vi "CRYUnflatten Limits.vi"(9 "Step Name":string, 11 "Unflatten Limits":string) -> (0 "Error?":bool, 2 "Limits":T1={"Name"="", "Tolerance"=2, "X Axis"=1, "Limits"=2, "Upper Limit"=[{100.0, 1.0}, {1000.0, 1.0}], "Align Ref"={1000.0, 0.0}, "Lower Limit"=[{100.0, -1.0}, {1000.0, -1.0}], "Y data"=1, "Y unit"="(und)", "Y dB ref"=1.0, "Curve Names"=[], "Y-Resolution"=1, "Type"=1, "x float"=FALSE, "X min-max-step"={"Limit X Offset Min"=0.9, "Limit X Offset Max"=1.1, "Limit X Offset Step Size"=1.01}, "magn/phase"=1, "Upper Limit Type"=0, "Lower Limit Type"=0, "Lim Curve axis up"=1, "Lim Curve axis lo"=1, "Data Selection Upper"=1, "Data Selection Lower"=1, "X-Resolution"=1, "Output failed point curves?"=FALSE, "X data"=1, "X unit"="(und)", "X dB ref"=1.0, "X-Y Graph Set-up"="", "Tab Value"=enum."Parameters", "Help"="", "X Up Val"=0.0, "Y Up Val"=0.0, "X Low Val"=0.0, "Y Low Val"=0.0, "Up Limit Val"=0.0, "Low Limit Val"=0.0, "bAdd DataName"=FALSE, "Custom Name"=""} {"X data" items=["dB", "Lin"]; "Data Selection Lower" items=["Single Values", "Curves", "Waveforms"]; "Data Selection Upper" items=["Single Values", "Curves", "Waveforms"]; "Lim Curve axis lo" items=["x", "y", "z"]; "Lim Curve axis up" items=["x", "y", "z"]; "Lower Limit Type" items=["User Defined", "Memory List"]; "Upper Limit Type" items=["User Defined", "Memory List"]; "Type" items=["Single Value", "Curve", "Waveforms", "Voltmeter"]; "Y data" items=["dB", "Lin"]; "Limits" items=["Upper Only", "Lower Only", "Upper & Lower"]; "X Axis" items=["Linear", "Logarithmic"]; "Tolerance" items=["Individual Points", "Absolute Limits", "Floating Limits", "Floating Data", "Aligned Limits", "Aligned Data"]}, 3 "Header info":T2={"Data type"="Data            ", "Version"=1, "Dimensions"=0})   [LabVIEW 2013]
uses:
  Typedef Control/CRYLimits.ctl
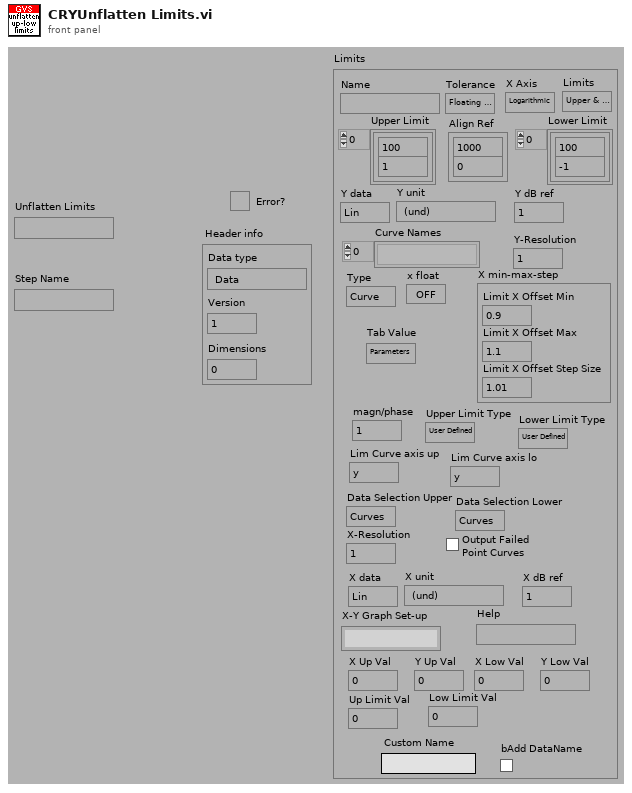
[diagram p1: front panel]
types:
  T1 = typedef "CRYLimits.ctl" = cluster{"Name":string, "Tolerance":u16, "X Axis":u16, "Limits":u16, "Upper Limit":cluster{dbl, dbl}[], "Align Ref":cluster{dbl, dbl}, "Lower Limit":cluster{dbl, dbl}[], "Y data":u16, "Y unit":string, "Y dB ref":dbl, "Curve Names":string[], "Y-Resolution":u8, "Type":u16, "x float":bool, "X min-max-step":cluster{"Limit X Offset Min":dbl, "Limit X Offset Max":dbl, "Limit X Offset Step Size":dbl}, "magn/phase":u16, "Upper Limit Type":u16, "Lower Limit Type":u16, "Lim Curve axis up":u16, "Lim Curve axis lo":u16, "Data Selection Upper":u16, "Data Selection Lower":u16, "X-Resolution":u8, "Output failed point curves?":bool, "X data":u16, "X unit":string, "X dB ref":dbl, "X-Y Graph Set-up":string, "Tab Value":enum32{"Data", "Parameters"}, "Help":string, "X Up Val":dbl, "Y Up Val":dbl, "X Low Val":dbl, "Y Low Val":dbl, "Up Limit Val":dbl, "Low Limit Val":dbl, "bAdd DataName":bool, "Custom Name":string}
  T2 = cluster{"Data type":string, "Version":u16, "Dimensions":u8}
  T3 = cluster{"Name":string, "Tolerance":u16, "X Axis":u16, "Limits":u16, "Upper Limit":cluster{dbl, dbl}[], "Align Ref":cluster{dbl, dbl}, "Lower Limit":cluster{dbl, dbl}[], "Y data":u16, "Y unit":string, "Y dB ref":dbl, "Curve Names":string[], "Y-Resolution":u8, "Type":u16, "x float":bool, "X min-max-step":cluster{"Limit X Offset Min":dbl, "Limit X Offset Max":dbl, "Limit X Offset Step Size":dbl}, "magn/phase":u16, "Upper Limit Type":u16, "Lower Limit Type":u16, "Lim Curve axis up":u16, "Lim Curve axis lo":u16, "Data Selection Upper":u16, "Data Selection Lower":u16, "X-Resolution":u8, "Output failed point curves?":bool, "X data":u16, "X unit":string, "X dB ref":dbl, "X-Y Graph Set-up":string, "Tab Value":enum32{"Data", "Parameters"}, "Help":string, "X Up Val":dbl, "Y Up Val":dbl, "X Low Val":dbl, "Y Low Val":dbl, "Up Limit Val":dbl, "Low Limit Val":dbl, "bAdd DataName":bool, "Custom Name":string}
  T4 = cluster{"unsigned byte array[0]":u8, "unsigned byte array[1]":u8, "unsigned byte array[2]":u8}
  T5 = cluster{"Name":string, "Tolerance":u16, "X Axis":u16, "Limits":u16, "Upper Limit":cluster{dbl, dbl}[], "Align Ref":cluster{dbl, dbl}, "Lower Limit":cluster{dbl, dbl}[], "Y data":u16, "Y unit":string, "Y dB ref":dbl, "Curve Names":string[], "Y-Resolution":u8, "Type":u16, "x float":bool, "X min-max-step":cluster{"Limit X Offset Min":dbl, "Limit X Offset Max":dbl, "Limit X Offset Step Size":dbl}, "magn/phase":u16, "Upper Limit Type":u16, "Lower Limit Type":u16, "Lim Curve axis up":u16, "Lim Curve axis lo":u16, "Data Selection Upper":u16, "Data Selection Lower":u16, "X-Resolution":u8, "Output failed point curves?":bool, "X data":u16, "X unit":string, "X dB ref":dbl, "X-Y Graph Set-up":string, "Tab Value":enum32{"Data", "Parameters", "Help"}}
  T6 = cluster{"Limit X Offset Min":dbl, "Limit X Offset Max":dbl, "Limit X Offset Step Size":dbl}
  T7 = cluster{"Name":string, "Tolerance":u16, "X Axis":u16, "Limits":u16, "Upper Limit":cluster{dbl, dbl}[], "Align Ref":cluster{dbl, dbl}, "Lower Limit":cluster{dbl, dbl}[], "Y data":u16, "Y unit":string, "Y dB ref":dbl, "Curve Names":string[], "Y-Resolution":u8, "Type":u16, "x float":bool, "X min-max-step":cluster{"Limit X Offset Min":dbl, "Limit X Offset Max":dbl, "Limit X Offset Step Size":dbl}, "magn/phase":u16, "Upper Limit Type":u16, "Lower Limit Type":u16, "Lim Curve axis up":u16, "Lim Curve axis lo":u16, "Data Selection Upper":u16, "Data Selection Lower":u16, "X-Resolution":u8, "Output failed point curves?":bool, "X data":u16, "X unit":string, "X dB ref":dbl, "X-Y Graph Set-up":string, "Tab Value":enum32{"Data", "Parameters"}, "Help":string}
  T8 = cluster{"Name":string, "Tolerance":u16, "X Axis":u16, "Limits":u16, "Upper Limit":cluster{dbl, dbl}[], "Align Ref":cluster{dbl, dbl}, "Lower Limit":cluster{dbl, dbl}[], "Y data":u16, "Y unit":string, "Y dB ref":dbl, "Curve Names":string[], "Y-Resolution":u8, "Type":u16, "x float":bool, "X min-max-step":cluster{"Limit X Offset Min":dbl, "Limit X Offset Max":dbl, "Limit X Offset Step Size":dbl}, "magn/phase":u16, "Upper Limit Type":u16, "Lower Limit Type":u16, "Lim Curve axis up":u16, "Lim Curve axis lo":u16, "Data Selection Upper":u16, "Data Selection Lower":u16, "X-Resolution":u8, "Output failed point curves?":bool, "X data":u16, "X unit":string, "X dB ref":dbl, "X-Y Graph Set-up":string, "Tab Value":enum32{"Data", "Parameters"}, "Help":string, "X Up Val":dbl, "Y Up Val":dbl, "X Low Val":dbl, "Y Low Val":dbl, "Up Limit Val":dbl, "Low Limit Val":dbl}
  T9 = cluster{"substring":string, u16, "unsigned byte array[2]":u8}
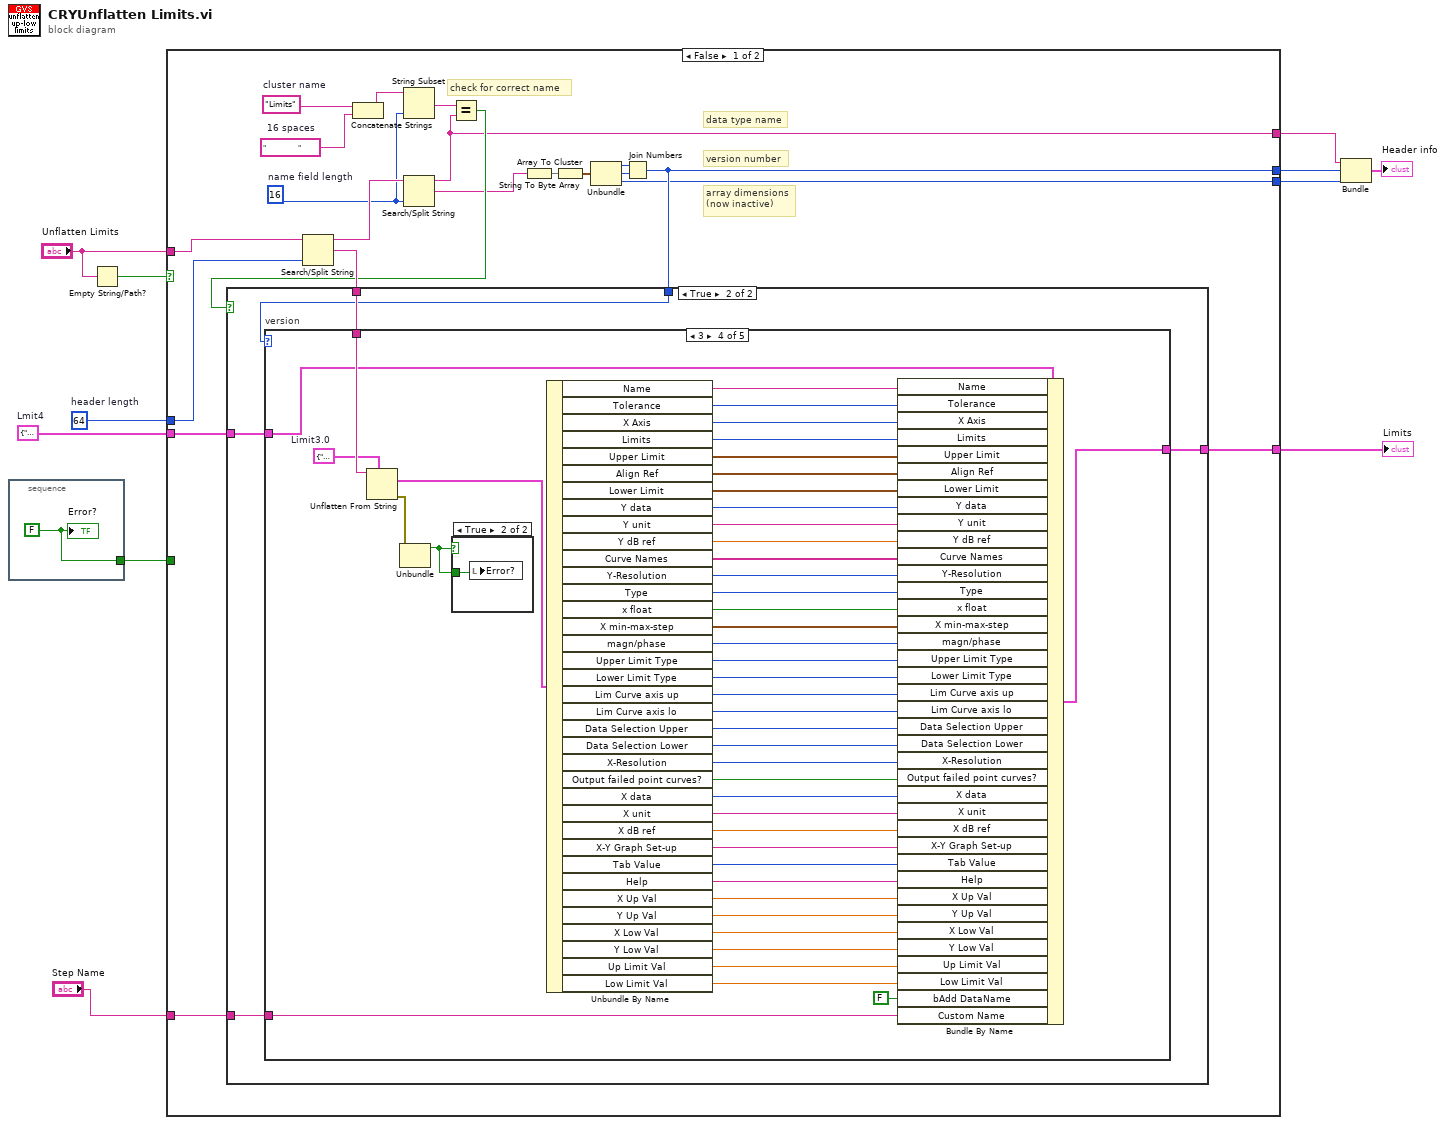
[diagram p0: block diagram]
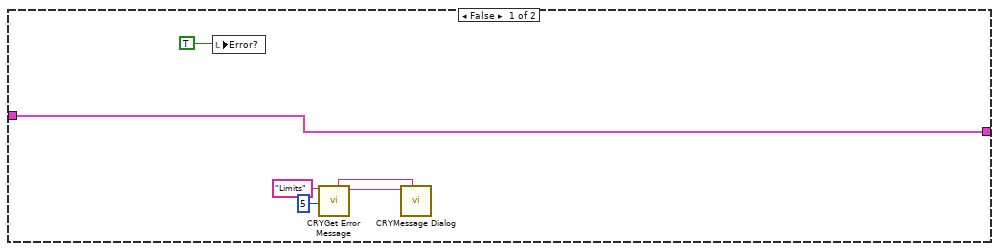
[diagram p2: hidden frame]
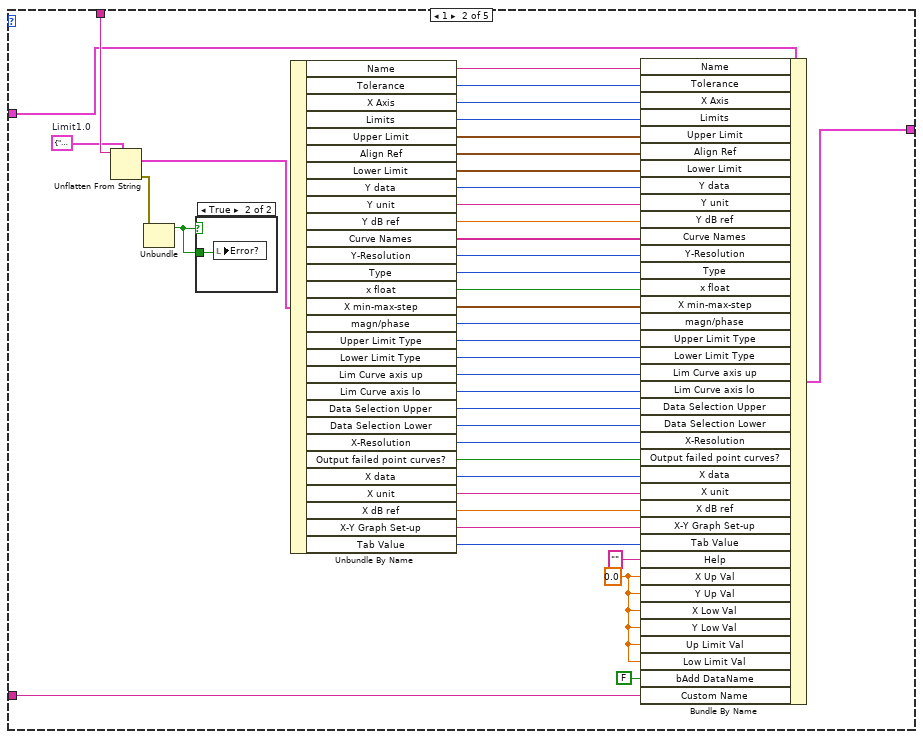
[diagram p4: hidden frame]
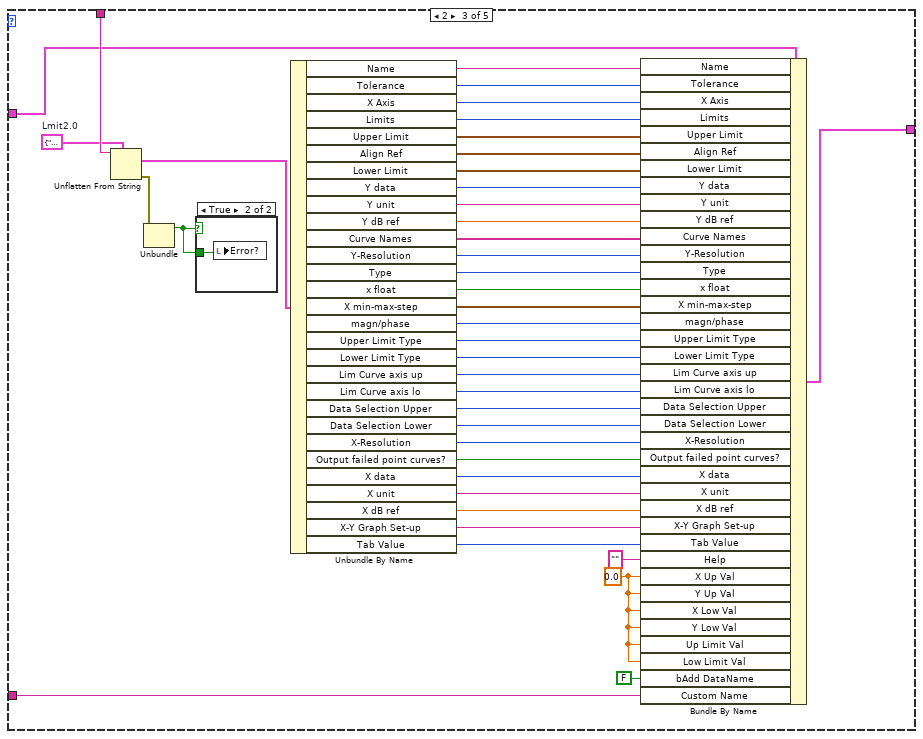
[diagram p6: hidden frame]
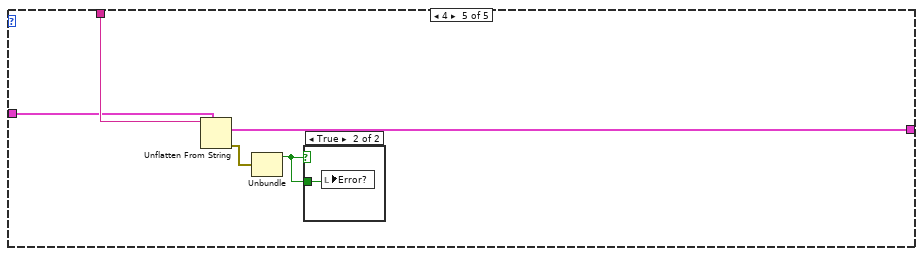
[diagram p9: hidden frame]
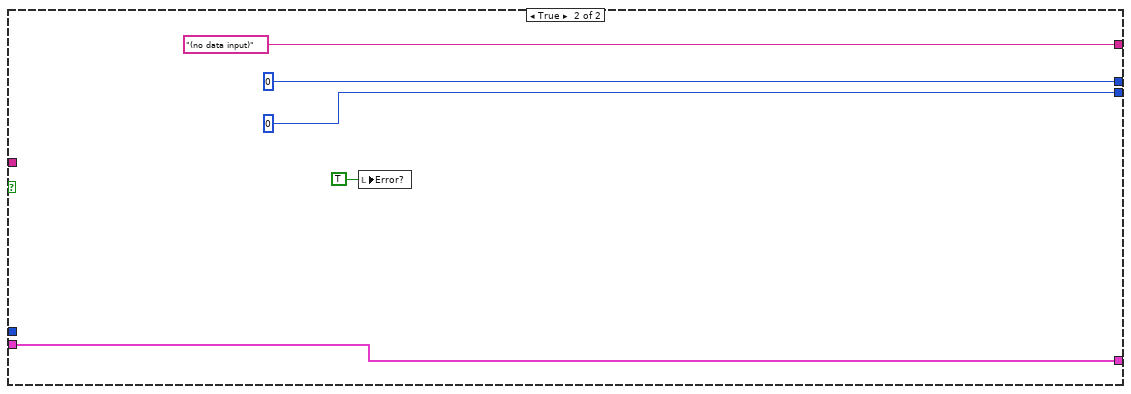
[diagram p11: hidden frame]
diagram:
  w3 = T3 {"Name"="", "Tolerance"=2, "X Axis"=1, "Limits"=2, "Upper Limit"=[{100.0, 1.0}, {1000.0, 1.0}], "Align Ref"={1000.0, 0.0}, "Lower Limit"=[{100.0, -1.0}, {1000.0, -1.0}], "Y data"=1, "Y unit"="(und)", "Y dB ref"=1.0, "Curve Names"=[], "Y-Resolution"=1, "Type"=1, "x float"=FALSE, "X min-max-step"={"Limit X Offset Min"=0.9, "Limit X Offset Max"=1.1, "Limit X Offset Step Size"=1.01}, "magn/phase"=1, "Upper Limit Type"=0, "Lower Limit Type"=0, "Lim Curve axis up"=1, "Lim Curve axis lo"=1, "Data Selection Upper"=1, "Data Selection Lower"=1, "X-Resolution"=1, "Output failed point curves?"=FALSE, "X data"=1, "X unit"="(und)", "X dB ref"=1.0, "X-Y Graph Set-up"="", "Tab Value"=enum."Parameters", "Help"="", "X Up Val"=0.0, "Y Up Val"=0.0, "X Low Val"=0.0, "Y Low Val"=0.0, "Up Limit Val"=0.0, "Low Limit Val"=0.0, "bAdd DataName"=FALSE, "Custom Name"=""}  # Lmit4
  w9 = 64  # header length
  n1 = stacked-sequence {
    tunnel: [w12] -> w4
    frame #0 {
      w12 = FALSE
      "Error?" <- w12
    }
  }
  n2 = Empty String/Path?(string/path="Unflatten Limits") -> (empty?=w10:bool)
  n3 = case shown="False" w10 {
    tunnel: "Unflatten Limits" -> [w33 _]
    tunnel: w9 -> [w27 _]
    tunnel: [w24 u16 0] -> w7
    tunnel: [w16 u8 0] -> w8
    tunnel: [w17 "(no data input)" ("substring")] -> w6
    tunnel: w4 -> [_ _]
    tunnel: [w15 w180] -> w2
    tunnel: w3 -> [w14 w180]
    tunnel: "Step Name" -> [w13 _]
    frame False {
      w21 = "                "  # 16 spaces
      w22 = "Limits"  # cluster name
      w19 = 16  # name field length
      # "check for correct name"
      # "array dimensions\n(now inactive)"
      # "version number"
      # "data type name"
      n4 = Search/Split String(string=w33, offset (0)=w27) -> (substring before match=w26:string, match + rest of string=w28:string)  [unwired: 2 out]
      n5 = Concatenate Strings(w22, w21) -> (w20:string)
      n6 = String Subset(string=w20, length (rest)=w19) -> (substring=w18:string)  [unwired: 1 out]
      n7 = Search/Split String(string=w26, offset (0)=w19) -> (substring before match=w17:string, match + rest of string=w23:string)  [unwired: 2 out]
      n8 = Equal?(x=w18, y=w17) -> (x = y?=w25:bool)
      n9 = String To Byte Array(string=w23) -> (unsigned byte array=w32:u8[])
      n10 = Array To Cluster(array=w32) -> (cluster=w31:T4)
      n11 = Unbundle(w31) -> ("unsigned byte array[0]"=w30:u8, "unsigned byte array[1]"=w29:u8, "unsigned byte array[2]"=w16:u8)
      n12 = Join Numbers(hi=w30, lo=w29) -> ((hi.lo)=w24:u16)
      n13 = case shown="True" w25 {
        tunnel: w28 -> [_ w44]
        tunnel: w24 -> [_ w43]
        tunnel: [w38 w42] -> w15
        tunnel: w14 -> [w38 w41]
        tunnel: w13 -> [_ w40]
        frame False {
          n14 = local write "Error?"(TRUE) -> ()
          n15 = call "CRYGet Error Message.vi"("Error No"=5 ("No"), "Kind"="Limits") -> ("Message"=w35:string, "Window Title"=w34:string)  [unwired: 4 in, 4 out]
          n16 = call "CRYMessage Dialog.vi"("Window Title"=w34, "Message Content"=w35) -> ()  [unwired: 8 in, 2 out]
        }
        frame True {
          n17 = case "version" shown="3" w43 {
            tunnel: w44 -> [_ w83 w124 w170 w178]
            tunnel: [w45 w50 w91 w138 w175] -> w42
            tunnel: w41 -> [w45 w81 w122 w168 w176]
            tunnel: w40 -> [_ w46 w87 w128 _]
            frame Default {
            }
            frame 1 {
              w49 = T5 {"Name"="", "Tolerance"=2, "X Axis"=1, "Limits"=2, "Upper Limit"=[{100.0, 1.0}, {1000.0, 1.0}], "Align Ref"={1000.0, 0.0}, "Lower Limit"=[{100.0, -1.0}, {1000.0, -1.0}], "Y data"=1, "Y unit"="(und)", "Y dB ref"=1.0, "Curve Names"=[], "Y-Resolution"=1, "Type"=1, "x float"=FALSE, "X min-max-step"={"Limit X Offset Min"=0.9, "Limit X Offset Max"=1.1, "Limit X Offset Step Size"=1.01}, "magn/phase"=1, "Upper Limit Type"=0, "Lower Limit Type"=0, "Lim Curve axis up"=1, "Lim Curve axis lo"=1, "Data Selection Upper"=1, "Data Selection Lower"=1, "X-Resolution"=1, "Output failed point curves?"=FALSE, "X data"=1, "X unit"="(und)", "X dB ref"=1.0, "X-Y Graph Set-up"="", "Tab Value"=enum."Data"}  # Limit1.0
              w48 = 0.0 ("X Up Val")
              n18 = Unflatten From String(type=w49, binary string=w83) -> (value=w82:T5, error out=w84:errorcluster)  [unwired: 1 in, 3 out]
              n19 = Unbundle(w84) -> ("status"=w85:bool)  [unwired: 2 out]
              n20 = case shown="True" w85 {
                tunnel: w85 -> [_ w86]
                frame False {
                }
                frame True {
                  n21 = local write "Error?"(w86) -> ()
                }
              }
              n22 = Unbundle By Name(w82) -> ("Name"=w80:string, "Tolerance"=w79:u16, "X Axis"=w78:u16, "Limits"=w77:u16, "Upper Limit"=w76:cluster{dbl, dbl}[], "Align Ref"=w75:cluster{dbl, dbl}, "Lower Limit"=w74:cluster{dbl, dbl}[], "Y data"=w73:u16, "Y unit"=w72:string, "Y dB ref"=w71:dbl, "Curve Names"=w70:string[], "Y-Resolution"=w69:u8, "Type"=w68:u16, "x float"=w67:bool, "X min-max-step"=w66:T6, "magn/phase"=w65:u16, "Upper Limit Type"=w64:u16, "Lower Limit Type"=w63:u16, "Lim Curve axis up"=w62:u16, "Lim Curve axis lo"=w61:u16, "Data Selection Upper"=w60:u16, "Data Selection Lower"=w59:u16, "X-Resolution"=w58:u8, "Output failed point curves?"=w57:bool, "X data"=w56:u16, "X unit"=w55:string, "X dB ref"=w54:dbl, "X-Y Graph Set-up"=w53:string, "Tab Value"=w52:enum32{"Data", "Parameters", "Help"})
              n23 = Bundle By Name(cluster=w81, "Name"=w80, "Tolerance"=w79, "X Axis"=w78, "Limits"=w77, "Upper Limit"=w76, "Align Ref"=w75, "Lower Limit"=w74, "Y data"=w73, "Y unit"=w72, "Y dB ref"=w71, "Curve Names"=w70, "Y-Resolution"=w69, "Type"=w68, "x float"=w67, "X min-max-step"=w66, "magn/phase"=w65, "Upper Limit Type"=w64, "Lower Limit Type"=w63, "Lim Curve axis up"=w62, "Lim Curve axis lo"=w61, "Data Selection Upper"=w60, "Data Selection Lower"=w59, "X-Resolution"=w58, "Output failed point curves?"=w57, "X data"=w56, "X unit"=w55, "X dB ref"=w54, "X-Y Graph Set-up"=w53, "Tab Value"=w52, "Help"="", "X Up Val"=w48, "Y Up Val"=w48, "X Low Val"=w48, "Y Low Val"=w48, "Up Limit Val"=w48, "Low Limit Val"=w48, "bAdd DataName"=FALSE, "Custom Name"=w46) -> (w50:T3)
            }
            frame 2 {
              w90 = T7 {"Name"="", "Tolerance"=2, "X Axis"=1, "Limits"=2, "Upper Limit"=[{100.0, 1.0}, {1000.0, 1.0}], "Align Ref"={1000.0, 0.0}, "Lower Limit"=[{100.0, -1.0}, {1000.0, -1.0}], "Y data"=1, "Y unit"="(und)", "Y dB ref"=1.0, "Curve Names"=[], "Y-Resolution"=1, "Type"=1, "x float"=FALSE, "X min-max-step"={"Limit X Offset Min"=0.9, "Limit X Offset Max"=1.1, "Limit X Offset Step Size"=1.01}, "magn/phase"=1, "Upper Limit Type"=0, "Lower Limit Type"=0, "Lim Curve axis up"=1, "Lim Curve axis lo"=1, "Data Selection Upper"=1, "Data Selection Lower"=1, "X-Resolution"=1, "Output failed point curves?"=FALSE, "X data"=1, "X unit"="(und)", "X dB ref"=1.0, "X-Y Graph Set-up"="", "Tab Value"=enum."Data", "Help"=""}  # Lmit2.0
              w89 = 0.0 ("X Up Val")
              n24 = Unflatten From String(type=w90, binary string=w124) -> (value=w123:T7, error out=w125:errorcluster)  [unwired: 1 in, 3 out]
              n25 = Unbundle(w125) -> ("status"=w126:bool)  [unwired: 2 out]
              n26 = case shown="True" w126 {
                tunnel: w126 -> [_ w127]
                frame False {
                }
                frame True {
                  n27 = local write "Error?"(w127) -> ()
                }
              }
              n28 = Unbundle By Name(w123) -> ("Name"=w121:string, "Tolerance"=w120:u16, "X Axis"=w119:u16, "Limits"=w118:u16, "Upper Limit"=w117:cluster{dbl, dbl}[], "Align Ref"=w116:cluster{dbl, dbl}, "Lower Limit"=w115:cluster{dbl, dbl}[], "Y data"=w114:u16, "Y unit"=w113:string, "Y dB ref"=w112:dbl, "Curve Names"=w111:string[], "Y-Resolution"=w110:u8, "Type"=w109:u16, "x float"=w108:bool, "X min-max-step"=w107:T6, "magn/phase"=w106:u16, "Upper Limit Type"=w105:u16, "Lower Limit Type"=w104:u16, "Lim Curve axis up"=w103:u16, "Lim Curve axis lo"=w102:u16, "Data Selection Upper"=w101:u16, "Data Selection Lower"=w100:u16, "X-Resolution"=w99:u8, "Output failed point curves?"=w98:bool, "X data"=w97:u16, "X unit"=w96:string, "X dB ref"=w95:dbl, "X-Y Graph Set-up"=w94:string, "Tab Value"=w93:enum32{"Data", "Parameters"})
              n29 = Bundle By Name(cluster=w122, "Name"=w121, "Tolerance"=w120, "X Axis"=w119, "Limits"=w118, "Upper Limit"=w117, "Align Ref"=w116, "Lower Limit"=w115, "Y data"=w114, "Y unit"=w113, "Y dB ref"=w112, "Curve Names"=w111, "Y-Resolution"=w110, "Type"=w109, "x float"=w108, "X min-max-step"=w107, "magn/phase"=w106, "Upper Limit Type"=w105, "Lower Limit Type"=w104, "Lim Curve axis up"=w103, "Lim Curve axis lo"=w102, "Data Selection Upper"=w101, "Data Selection Lower"=w100, "X-Resolution"=w99, "Output failed point curves?"=w98, "X data"=w97, "X unit"=w96, "X dB ref"=w95, "X-Y Graph Set-up"=w94, "Tab Value"=w93, "Help"="", "X Up Val"=w89, "Y Up Val"=w89, "X Low Val"=w89, "Y Low Val"=w89, "Up Limit Val"=w89, "Low Limit Val"=w89, "bAdd DataName"=FALSE, "Custom Name"=w87) -> (w91:T3)
            }
            frame 3 {
              w137 = T8 {"Name"="", "Tolerance"=2, "X Axis"=1, "Limits"=2, "Upper Limit"=[{100.0, 1.0}, {1000.0, 1.0}], "Align Ref"={1000.0, 0.0}, "Lower Limit"=[{100.0, -1.0}, {1000.0, -1.0}], "Y data"=1, "Y unit"="(und)", "Y dB ref"=1.0, "Curve Names"=[], "Y-Resolution"=1, "Type"=1, "x float"=FALSE, "X min-max-step"={"Limit X Offset Min"=0.9, "Limit X Offset Max"=1.1, "Limit X Offset Step Size"=1.01}, "magn/phase"=1, "Upper Limit Type"=0, "Lower Limit Type"=0, "Lim Curve axis up"=1, "Lim Curve axis lo"=1, "Data Selection Upper"=1, "Data Selection Lower"=1, "X-Resolution"=1, "Output failed point curves?"=FALSE, "X data"=1, "X unit"="(und)", "X dB ref"=1.0, "X-Y Graph Set-up"="", "Tab Value"=enum."Parameters", "Help"="", "X Up Val"=0.0, "Y Up Val"=0.0, "X Low Val"=0.0, "Y Low Val"=0.0, "Up Limit Val"=0.0, "Low Limit Val"=0.0}  # Limit3.0
              n30 = Unflatten From String(type=w137, binary string=w170) -> (value=w169:T8, error out=w171:errorcluster)  [unwired: 1 in, 3 out]
              n31 = Unbundle(w171) -> ("status"=w172:bool)  [unwired: 2 out]
              n32 = case shown="True" w172 {
                tunnel: w172 -> [_ w173]
                frame False {
                }
                frame True {
                  n33 = local write "Error?"(w173) -> ()
                }
              }
              n34 = Unbundle By Name(w169) -> ("Name"=w167:string, "Tolerance"=w166:u16, "X Axis"=w165:u16, "Limits"=w164:u16, "Upper Limit"=w163:cluster{dbl, dbl}[], "Align Ref"=w162:cluster{dbl, dbl}, "Lower Limit"=w161:cluster{dbl, dbl}[], "Y data"=w160:u16, "Y unit"=w159:string, "Y dB ref"=w158:dbl, "Curve Names"=w157:string[], "Y-Resolution"=w156:u8, "Type"=w155:u16, "x float"=w154:bool, "X min-max-step"=w153:T6, "magn/phase"=w152:u16, "Upper Limit Type"=w151:u16, "Lower Limit Type"=w150:u16, "Lim Curve axis up"=w149:u16, "Lim Curve axis lo"=w148:u16, "Data Selection Upper"=w147:u16, "Data Selection Lower"=w146:u16, "X-Resolution"=w145:u8, "Output failed point curves?"=w144:bool, "X data"=w143:u16, "X unit"=w142:string, "X dB ref"=w141:dbl, "X-Y Graph Set-up"=w140:string, "Tab Value"=w139:enum32{"Data", "Parameters"}, "Help"=w136:string, "X Up Val"=w135:dbl, "Y Up Val"=w134:dbl, "X Low Val"=w133:dbl, "Y Low Val"=w132:dbl, "Up Limit Val"=w131:dbl, "Low Limit Val"=w130:dbl)
              n35 = Bundle By Name(cluster=w168, "Name"=w167, "Tolerance"=w166, "X Axis"=w165, "Limits"=w164, "Upper Limit"=w163, "Align Ref"=w162, "Lower Limit"=w161, "Y data"=w160, "Y unit"=w159, "Y dB ref"=w158, "Curve Names"=w157, "Y-Resolution"=w156, "Type"=w155, "x float"=w154, "X min-max-step"=w153, "magn/phase"=w152, "Upper Limit Type"=w151, "Lower Limit Type"=w150, "Lim Curve axis up"=w149, "Lim Curve axis lo"=w148, "Data Selection Upper"=w147, "Data Selection Lower"=w146, "X-Resolution"=w145, "Output failed point curves?"=w144, "X data"=w143, "X unit"=w142, "X dB ref"=w141, "X-Y Graph Set-up"=w140, "Tab Value"=w139, "Help"=w136, "X Up Val"=w135, "Y Up Val"=w134, "X Low Val"=w133, "Y Low Val"=w132, "Up Limit Val"=w131, "Low Limit Val"=w130, "bAdd DataName"=FALSE, "Custom Name"=w128) -> (w138:T3)
            }
            frame 4 {
              n36 = Unflatten From String(type=w176, binary string=w178) -> (value=w175:T3, error out=w174:errorcluster)  [unwired: 1 in, 3 out]
              n37 = Unbundle(w174) -> ("status"=w177:bool)  [unwired: 2 out]
              n38 = case shown="True" w177 {
                tunnel: w177 -> [_ w179]
                frame False {
                }
                frame True {
                  n39 = local write "Error?"(w179) -> ()
                }
              }
            }
          }
        }
      }
    }
    frame True {
      n40 = local write "Error?"(TRUE ("Error?")) -> ()
    }
  }
  "Limits" <- w2
  n41 = Bundle("substring"=w6, w7, "unsigned byte array[2]"=w8) -> (→"Header info":T9)  [unwired: 1 out]
